vi "Measurement UI.vi"() -> ()   [LabVIEW 2021, in "Tree.lvlib"]
uses:
  Tree.lvlib
panel:
  out "State":bool[](array[boolean])
  in  "randomise tree":bool
  in  "restore state":bool
  in  "save state":bool
  in  "Tree":string(tree)="child 8"
  # "Source: https://forums.ni.com/t5/Example-Code/LabVIEW-Tree-Control-Save-and-Restore-the-Status-of-a-Heirarchy/ta-p/3506610"
  # "Save / Recall of hierarchy tree state"
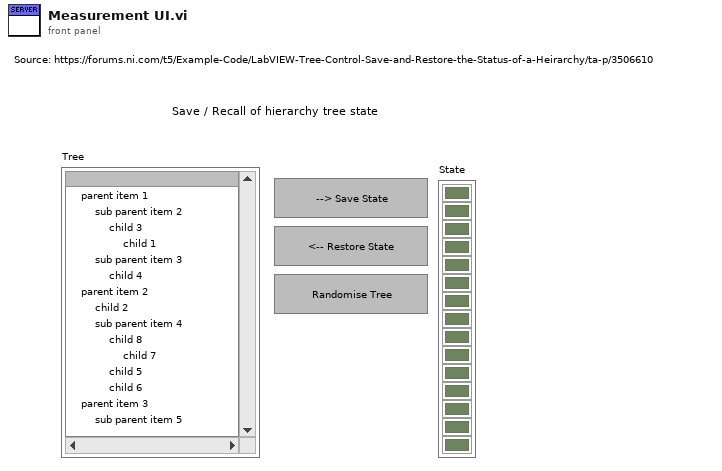
[diagram p1: front panel]
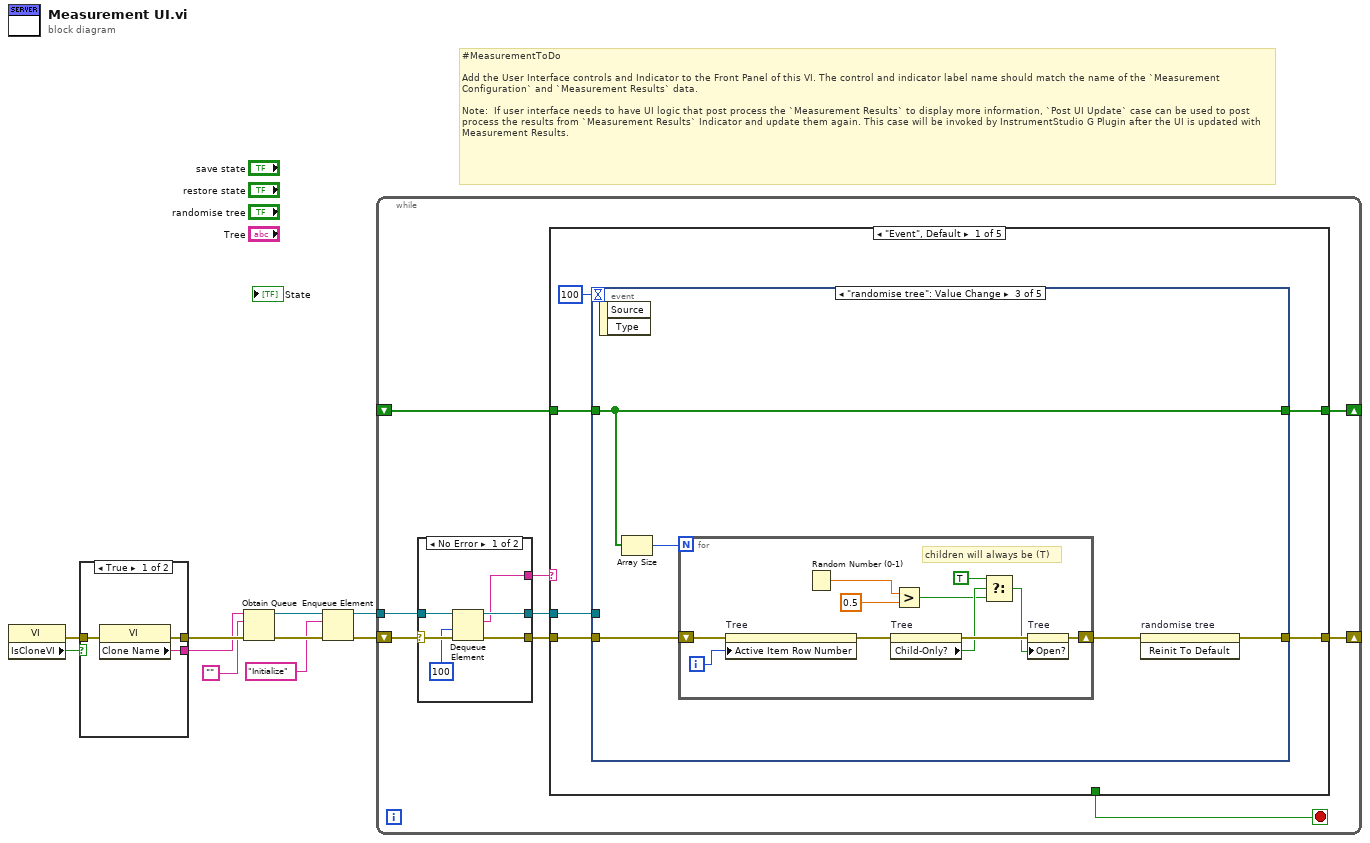
[diagram p0: block diagram]
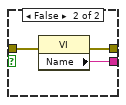
[diagram p2: hidden frame]
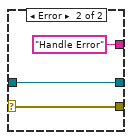
[diagram p3: hidden frame]
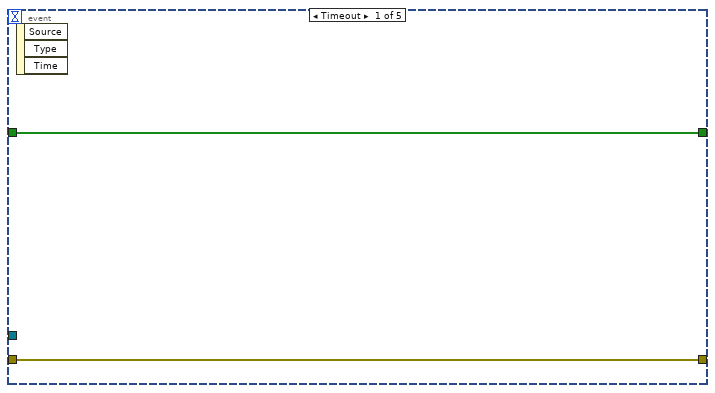
[diagram p4: hidden frame]
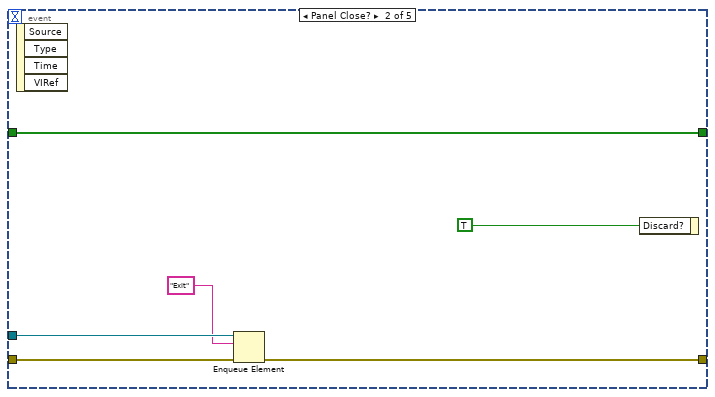
[diagram p5: hidden frame]
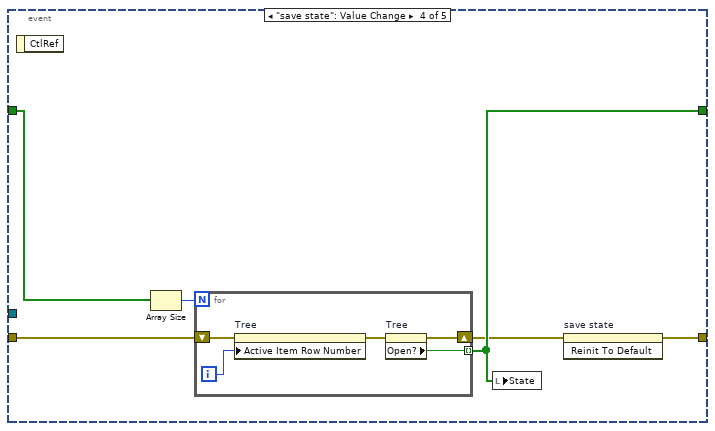
[diagram p6: hidden frame]
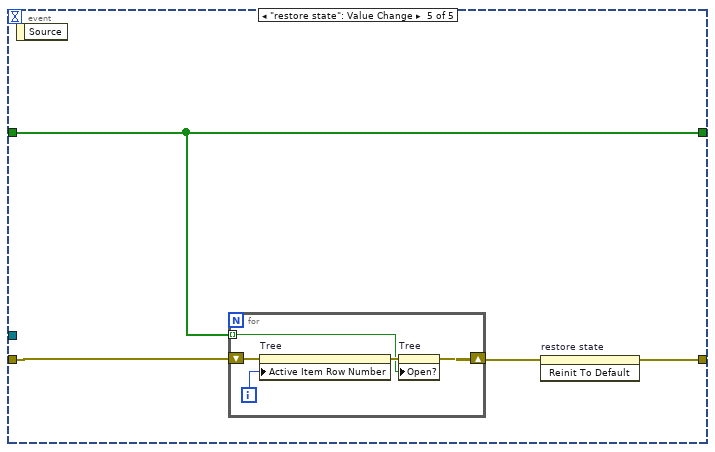
[diagram p7: hidden frame]
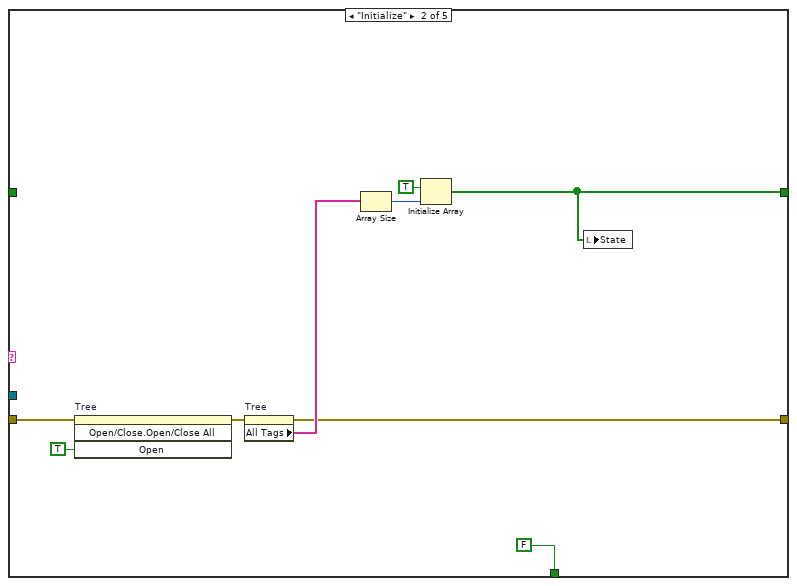
[diagram p8: hidden frame]
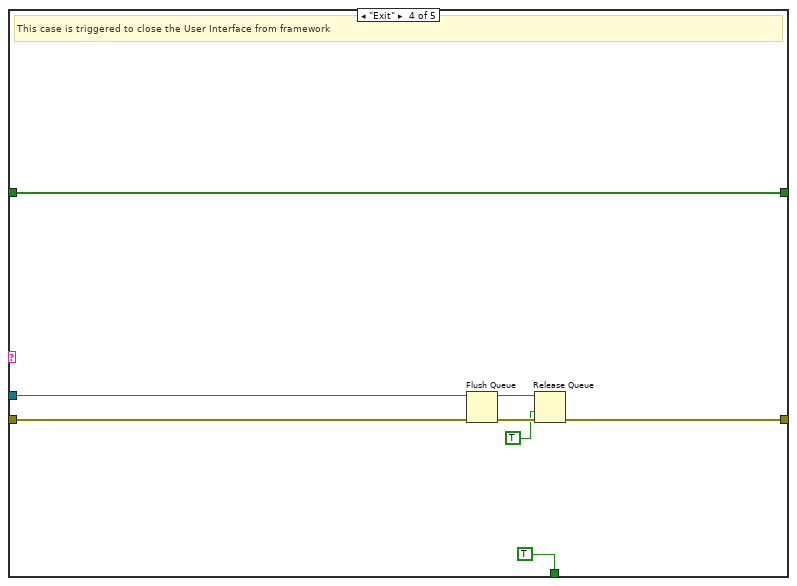
[diagram p10: hidden frame]
diagram:
  # "#MeasurementToDo  \n\nAdd the User Interface controls and Indicator to the Front Panel of this VI. The control and indicator label name should match the name of the `Measurement Configuration` and `Measurement Results` data.\n\nNote:  If user interface needs to have UI logic that post process the `Measurement Results` to display more information, `Post UI Update` case can be used to post process the results from `Measurement Results` Indicator and update them again. This case will be invoked by InstrumentStudio G Plugin after the UI is updated with Measurement Results."
  n1 = property class="VI"() -> (error out=w1:errorcluster, "IsCloneVI"=w2:bool)  [unwired: 2 in, 1 out]
  n2 = case shown="True" w2 {
    tunnel: [w13 w16] -> w10
    tunnel: [w12 w15] -> w9
    tunnel: w1 -> [w11 w14]
    frame True {
      n3 = property class="VI"(error in=w11) -> (error out=w13:errorcluster, "Clone Name"=w12:string)  [unwired: 1 in, 1 out]
    }
    frame False {
      n4 = property class="VI"(error in=w14) -> (error out=w16:errorcluster, "Name"=w15:string)  [unwired: 1 in, 1 out]
    }
  }
  n5 = Obtain Queue(name (unnamed)=w9, element data type="", error in (no error)=w10) -> (queue out=w6:refnum<queue>, error out=w8:errorcluster)  [unwired: 2 in, 1 out]
  n6 = Enqueue Element(queue=w6, element="Initialize", error in (no error)=w8) -> (queue out=w5:refnum<queue>, error out=w7:errorcluster)  [unwired: 1 in, 1 out]
  n7 = while {
    shift-right: [w20] -> _
    shift-left: w7 -> [w25]
    tunnel: w5 -> [w23]
    shift-right: [w18] -> _
    shift-left: _ -> [w17]
    stop <- w19 stop-if-true
    n8 = case shown="No Error" w25 {
      selector: w25 -> [w31 w34]
      tunnel: [w30 w34] -> w24
      tunnel: w23 -> [w29 w33]
      tunnel: [w28 w33] -> w22
      tunnel: [w27 "Handle Error"] -> w21
      frame No Error {
        n9 = Dequeue Element(queue=w29, timeout in ms (-1)=100, error in (no error)=w31) -> (queue out=w28:refnum<queue>, element=w27:string, error out=w30:errorcluster)  [unwired: 1 out]
      }
      frame Error {
      }
    }
    n10 = case shown="\"Event\", Default" w21 {
      tunnel: w24 -> [w39 w87 w95 w103 w105]
      tunnel: w22 -> [w37 _ _ w101 _]
      tunnel: [w40 w85 w95 w98 w105] -> w20
      tunnel: [_ FALSE _ TRUE _] -> w19
      tunnel: [w35 w86 w94 w96 w104] -> w18
      tunnel: w17 -> [w36 _ w94 w96 w104]
      frame "Event", Default {
        n11 = event shown="[2] \"randomise tree\": Value Change" {
          selector: _ -> [_ _ _ _ _]
          dyn-events: _ -> [_ _ _ _ _]
          timeout: 100 -> [_ _ _ _ _]
          tunnel: [w42 w46 w49 w65 w76] -> w40
          tunnel: w39 -> [w42 w47 w51 w69 w79]
          tunnel: w37 -> [_ w45 _ _ _]
          tunnel: w36 -> [w41 w43 w52 w68 w78]
          tunnel: [w41 w43 w52 w67 w78] -> w35
          event Timeout {
            n12 = event-data() -> ()  [unwired: 1 in, 3 out]
          }
          event Panel Close? {
            n13 = event-data() -> ()  [unwired: 1 in, 4 out]
            n14 = Enqueue Element(queue=w45, element="Exit", error in (no error)=w47) -> (error out=w46:errorcluster)  [unwired: 1 in, 2 out]
            n15 = event-data("Discard?"=TRUE) -> ()  [unwired: 1 in, 1 out]
          }
          event "randomise tree": Value Change {
            n16 = event-data() -> ()  [unwired: 1 in, 2 out]
            n17 = Array Size(array=w52) -> (size(s)=w53:i32)
            n18 = for {
              N: w53 -> [_]
              shift-right: [w60] -> w50
              shift-left: w51 -> [w62]
              i -> [w61]
              # "children will always be (T)"
              n19 = property on="Tree" class="Tree (strict)"(error in=w62, "Active Item Row Number"=w61) -> (error out=w59:errorcluster)  [unwired: 1 in, 1 out]
              n20 = Random Number (0-1)() -> (number: 0 to 1=w64:dbl)
              n21 = property on="Tree" class="Tree (strict)"(error in=w59) -> (error out=w58:errorcluster, "Child-Only?"=w57:bool)  [unwired: 1 in, 1 out]
              n22 = Greater?(x=w64, y=0.5) -> (0:w56:bool)
              n23 = Select(t=TRUE, s=w57, f=w56) -> (s? t:f=w54:bool)
              n24 = property on="Tree" class="Tree (strict)"(error in=w58, "Open?"=w54) -> (error out=w60:errorcluster)  [unwired: 1 in, 1 out]
            }
            n25 = invoke on="randomise tree" class="Bool" method="Reinit To Default"(error in=w50) -> (error out=w49:errorcluster)  [unwired: 2 in, 2 out]
          }
          event "save state": Value Change {
            n26 = event-data() -> ()  [unwired: 1 in, 1 out]
            n27 = Array Size(array=w68) -> (size(s)=w70:i32)
            n28 = for {
              N: w70 -> [_]
              tunnel: [w73] -> w67 mode=indexing
              shift-right: [w71] -> w66
              shift-left: w69 -> [w72]
              i -> [w75]
              n29 = property on="Tree" class="Tree (strict)"(error in=w72, "Active Item Row Number"=w75) -> (error out=w74:errorcluster)  [unwired: 1 in, 1 out]
              n30 = property on="Tree" class="Tree (strict)"(error in=w74) -> (error out=w71:errorcluster, "Open?"=w73:bool)  [unwired: 1 in, 1 out]
            }
            n31 = local write "State"(w67) -> ()
            n32 = invoke on="save state" class="Bool" method="Reinit To Default"(error in=w66) -> (error out=w65:errorcluster)  [unwired: 2 in, 2 out]
          }
          event "restore state": Value Change {
            n33 = event-data() -> ()  [unwired: 1 in, 1 out]
            n34 = for {
              tunnel: w78 -> [w82] mode=indexing
              shift-right: [w80] -> w77
              shift-left: w79 -> [w81]
              i -> [w84]
              n35 = property on="Tree" class="Tree (strict)"(error in=w81, "Active Item Row Number"=w84) -> (error out=w83:errorcluster)  [unwired: 1 in, 1 out]
              n36 = property on="Tree" class="Tree (strict)"(error in=w83, "Open?"=w82) -> (error out=w80:errorcluster)  [unwired: 1 in, 1 out]
            }
            n37 = invoke on="restore state" class="Bool" method="Reinit To Default"(error in=w77) -> (error out=w76:errorcluster)  [unwired: 2 in, 2 out]
          }
        }
      }
      frame "Initialize" {
        n38 = invoke on="Tree" class="Tree (strict)" method="Open/Close.Open/Close All"(error in=w87, "Open"=TRUE ("Open?")) -> (error out=w89:errorcluster)  [unwired: 2 in, 3 out]
        n39 = property on="Tree" class="Tree (strict)"(error in=w89) -> (error out=w85:errorcluster, "All Tags"=w90:string[])  [unwired: 1 in, 1 out]
        n40 = Array Size(array=w90) -> (size(s)=w91:i32)
        n41 = Initialize Array(TRUE, w91) -> (w86:bool[])
        n42 = local write "State"(w86) -> ()
      }
      frame "Post UI Update" {
        # "This case will be triggered, after framework updates the User interface with result values."
      }
      frame "Exit" {
        # "This case is triggered to close the User Interface from framework"
        n43 = Flush Queue(queue=w101, error in (no error)=w103) -> (queue out=w100:refnum<queue>, error out=w99:errorcluster)  [unwired: 1 out]
        n44 = Release Queue(queue=w100, force destroy? (F)=TRUE, error in (no error)=w99) -> (error out=w98:errorcluster)  [unwired: 2 out]
      }
      frame "Handle Error" {
      }
    }
  }
